vi "Target Analog Read PXIe 6363.vi"(11 "task/channels in":refnum<k21>) -> (0 "GRF Z (V)":dbl, 2 "Encoder Voltage B":dbl, 3 "Encoder Voltage A":dbl, 4 "Vicon Log Trigger":dbl)   [LabVIEW 2018, in "COBRA Measurement and Filtering Library.lvlib"]
uses:
  COBRA Measurement and Filtering Library.lvlib
  <vilib>/DAQmx/read.llb/DAQmx Read (Analog 1D DBL NChan 1Samp).vi
  <vilib>/DAQmx/miscellaneous.llb/DAQmx Fill In Error Info.vi
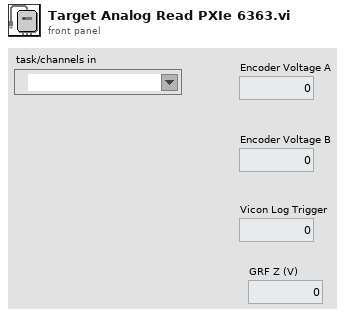
[diagram p1: front panel]
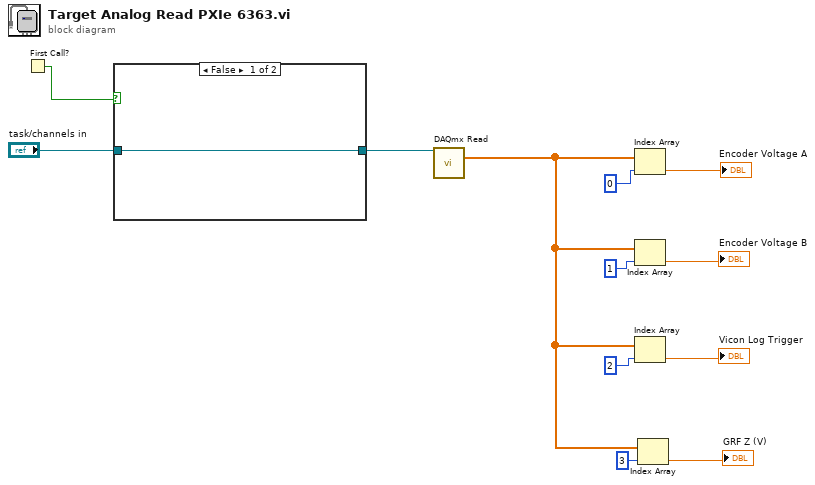
[diagram p0: block diagram]
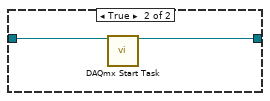
[diagram p2: hidden frame]
diagram:
  n1 = First Call?() -> (First Call?: T/F=w4:bool)
  n2 = case shown="False" w4 {
    tunnel: "task/channels in" -> [w13 w15]
    tunnel: [w13 w14] -> w9
    frame False {
    }
    frame True {
      n3 = call <vilib>:"DAQmx Start Task.vi"("task/channels in"=w15) -> ("task out"=w14:refnum<k21>)  [unwired: 13 in, 1 out]
    }
  }
  n4 = call-poly <vilib>:"DAQmx Read.vi"("task/channels in"=w9) -> ("data"=w3:dbl[])  [unwired: 12 in, 2 out]
  n5 = Index Array(array=w3, index=0) -> (element=→"Encoder Voltage A":dbl)
  n6 = Index Array(array=w3, index=1) -> (element=→"Encoder Voltage B":dbl)
  n7 = Index Array(array=w3, index=2) -> (element=→"Vicon Log Trigger":dbl)
  n8 = Index Array(array=w3, index=3) -> (element=→"GRF Z (V)":dbl)
